vi "A33ConfigureTrigger.vi"(0 "VISA resource name":refnum<visa-resource-name>, 1 "Trigger Source (0: Immediate)":u16(ring)=2 items=["Immediate (Burst period)", "Timer", "External", "Software Trigger Function"], 2 "Trigger Level (0.9-3.8V)":dbl=2.0 format="%#_12g", 5 "Channel (1: Channel1)":u16(ring)=1 items=["Channel1"=1, "Channel2"=2], 7 "Int period (1 s)":dbl=1.0 format="%#_12g", 9 "Delay (0 s)":dbl format="%#_12g", 11 "error in (no error)":errorcluster, 12 "Trigger Slope (0: Positive)":u16(ring) items=["Positive", "Negative"]) -> (4 "VISA resource name out":refnum<visa-resource-name>, 15 "error out":errorcluster)   [LabVIEW 2022 SP3]
doc: "Configures the trigger source for triggering sweeps.\n\n<B>Note:</B> Use this VI only with other low-level VIs. The high-level VIs automatically incorporate this functionality. This VI does not check the instrument status. If you want to check the instrument status, call the Error Query VI at the conclusion of your sweep operation."
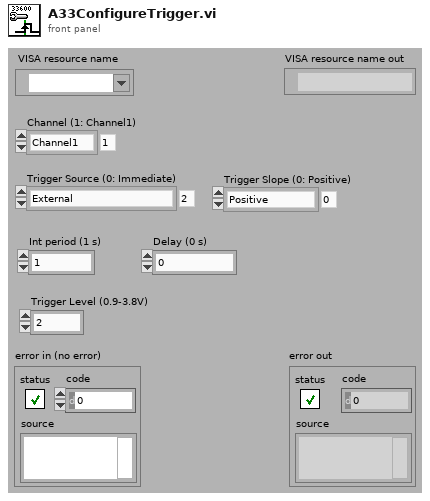
[diagram p1: front panel]
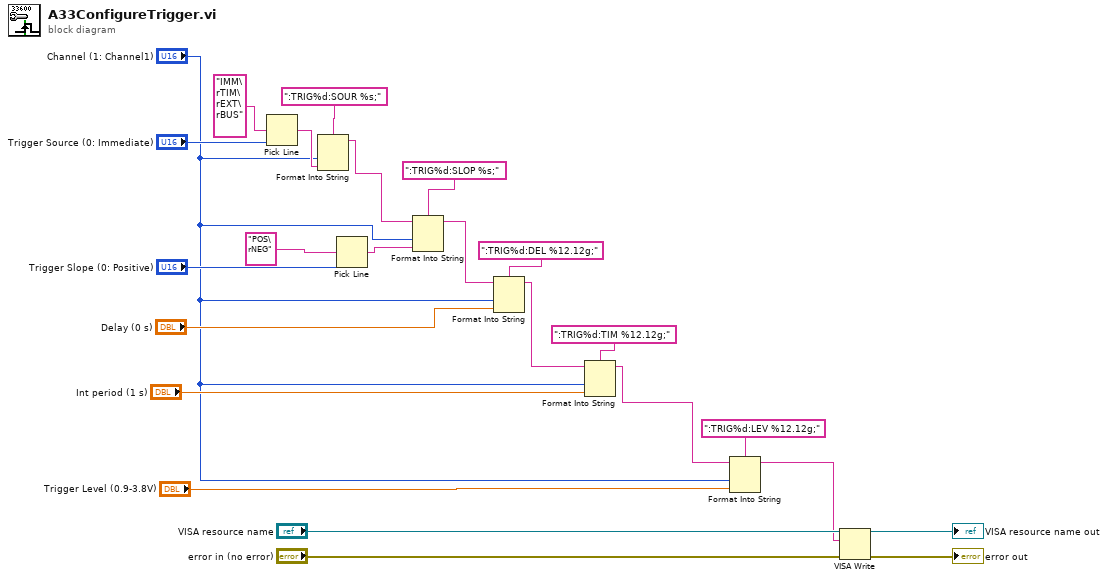
[diagram p0: block diagram]
diagram:
  n1 = Pick Line(multi-line string="IMM\rTIM\rEXT\rBUS", line index="Trigger Source (0: Immediate)") -> (output string=w21:string)  [unwired: 1 in]
  n2 = Format Into String(format string=":TRIG%d:SOUR %s;", "Channel (1: Channel1)", w21) -> (resulting string=w7:string)  [unwired: 2 in, 1 out]
  n3 = Pick Line(multi-line string="POS\rNEG", line index="Trigger Slope (0: Positive)") -> (output string=w8:string)  [unwired: 1 in]
  n4 = Format Into String(format string=":TRIG%d:SLOP %s;", initial string=w7, "Channel (1: Channel1)", w8) -> (resulting string=w4:string)  [unwired: 1 in, 1 out]
  n5 = Format Into String(format string=":TRIG%d:DEL %12.12g;", initial string=w4, "Channel (1: Channel1)", "Delay (0 s)") -> (resulting string=w5:string)  [unwired: 1 in, 1 out]
  n6 = Format Into String(format string=":TRIG%d:TIM %12.12g;", initial string=w5, "Channel (1: Channel1)", "Int period (1 s)") -> (resulting string=w10:string)  [unwired: 1 in, 1 out]
  n7 = Format Into String(format string=":TRIG%d:LEV %12.12g;", initial string=w10, "Channel (1: Channel1)", "Trigger Level (0.9-3.8V)") -> (resulting string=w11:string)  [unwired: 1 in, 1 out]
  n8 = VISA Write(VISA resource name="VISA resource name", write buffer=w11, error in (no error)="error in (no error)") -> (VISA resource name out=→"VISA resource name out":refnum<visa-resource-name>, error out=→"error out":errorcluster)  [unwired: 1 out]
